vi "ROI Entry Screen.vi"() -> ()   [LabVIEW 2017]
uses:
  Typedefs/Line draw mode.ctl
  Typedefs/Top level VI states.ctl
  ROI Entry screen/Typedefs/ROI move buttons.ctl
  ROI Entry screen/Typedefs/ROI move mode.ctl
  Typedefs/Offsets cluster.ctl
  Typedefs/ROI management FG states.ctl
  ROI Entry screen/SubVIs/Automatic POI detection/Typedefs/Duplicate POI function enum.ctl
  Typedefs/Read Write Enum.ctl
  ROI Entry screen/Typedefs/ROI entry screen ctrl refs cluster.ctl
  Global Variables/General Globals.vi
  User profiles code/Globals/gl_UsrProfiles globals.vi
  ROI Entry screen/Globals/gl_ROI Entry UI globals.vi
  ROI Entry screen/Typedefs/ROI input mode.ctl
panel:
  out "Current ROI Type":string
  out "AOL Z ind. (um)":dbl caption="Motor Z" format="AOL Z   =  %#_g µm"
  in  "Load Reference Image":bool
  out "# POI":i32 format="%.0f ROI"
  in  "Max Z Proj":bool
  out "ROI":T1
  out "Number of lines left":i32 format="%.0f number of lines left"
  in  "Palette Type":T2(ring)
  out "Zplane ind":i32 caption="Z-Plane" format="Z-Plane %.0f"
  in  "Z-Plane Selector":i32(c297)=7
  out "Image Display":T3(plugin-control)
  out "Motor Z ind. (um)":dbl caption="Motor Z" format="Motor Z = %#_g µm"
  out "# of planes":i32 format="# of Planes = %.0f"
  in  "Intensity slider":cluster{i16, i16}(slide)={0, 4095} caption="Intensity" scale=0.0..4095.0
  in  "Z-stack folder path":path caption="Experiment folder path"
  in  "Channel":enum16{"Green", "Red"}(ring)
  in  "Enable cool-down time":bool caption="Enable stimulus"
  in  "Cool-down time (s)":dbl caption="Cool-down time" min=0.0 max=60.0 step=0.05 format="%#.2f s"
  in  "Enable funct. stimulus":bool caption="Enable stimulus"
  in  "Funct stim.trig.delay (sec)":dbl=0.5 caption="Stimulus trigger delay" min=0.0 max=60.0 step=0.001 format="%#.3fs"
  in  "ROI move mode":T4
  in  "ROI offset arrows":T5
  in  "Trial Length (sec)":dbl=1.0 caption="Trial Length" min=0.05 max=60.0 step=1.0 format="%#.3f s"
  in  "Arb Plane Entry":bool caption="Load\nolder\nPOI"
  in  "Load ROI File":bool caption="Load\nolder\nPOI"
  in  "POI Density":dbl(slide) scale=0.01..1.0
  in  "Auto Generate":bool
  in  "Equal size":bool=TRUE
  in  "Whole plane":bool
  in  "Zoom":dbl=1.0 min=0.001 max=10.0 step=0.1 format="%#.2f x"
  out "Next State":T6=enum."Live Imaging-START"
  in  "Scan dwell time per pixel (us)":dbl=0.1 caption="Scan dwell time\nper pixel (us)" min=0.05 max=20.0 step=0.01 format="%.2f"
  in  "POI dwell time (us)":dbl=4.0 caption="POI dwell time" min=0.05 max=20.0 format="%_3g µs"
  in  "Live Imaging":bool
  in  "Acquisition":bool
  in  "Line Mode":T7=enum."Orthogonal"
  in  "Number of Trials":u16=1 min=1 max=1000 format="%.0f trials"
  in  "Wavelength (nm)":dbl=920.0 caption="Wavelength" min=800.0 max=1080.0 step=1.0 format="%#_g nm"
  in  "Done/Close":bool
  in  "Clear Last":bool
  in  "Clear All":bool
  in  "POISelect Array":cluster{"System Array":dbl[], "Boolean":bool}[](array[cluster])
  in  "Step size (µm)":u8(slide)=1 min=1 max=100 step=1 scale=1.0..30.0
  # "ROI Removal"
  # "ROI Input"
  # "ROI AutoGen"
  # "Min"
  # "Max"
  # "Stimulus trigger delay"
  # "Cool-down time"
  # "ROI Offset"
  # "Settings"
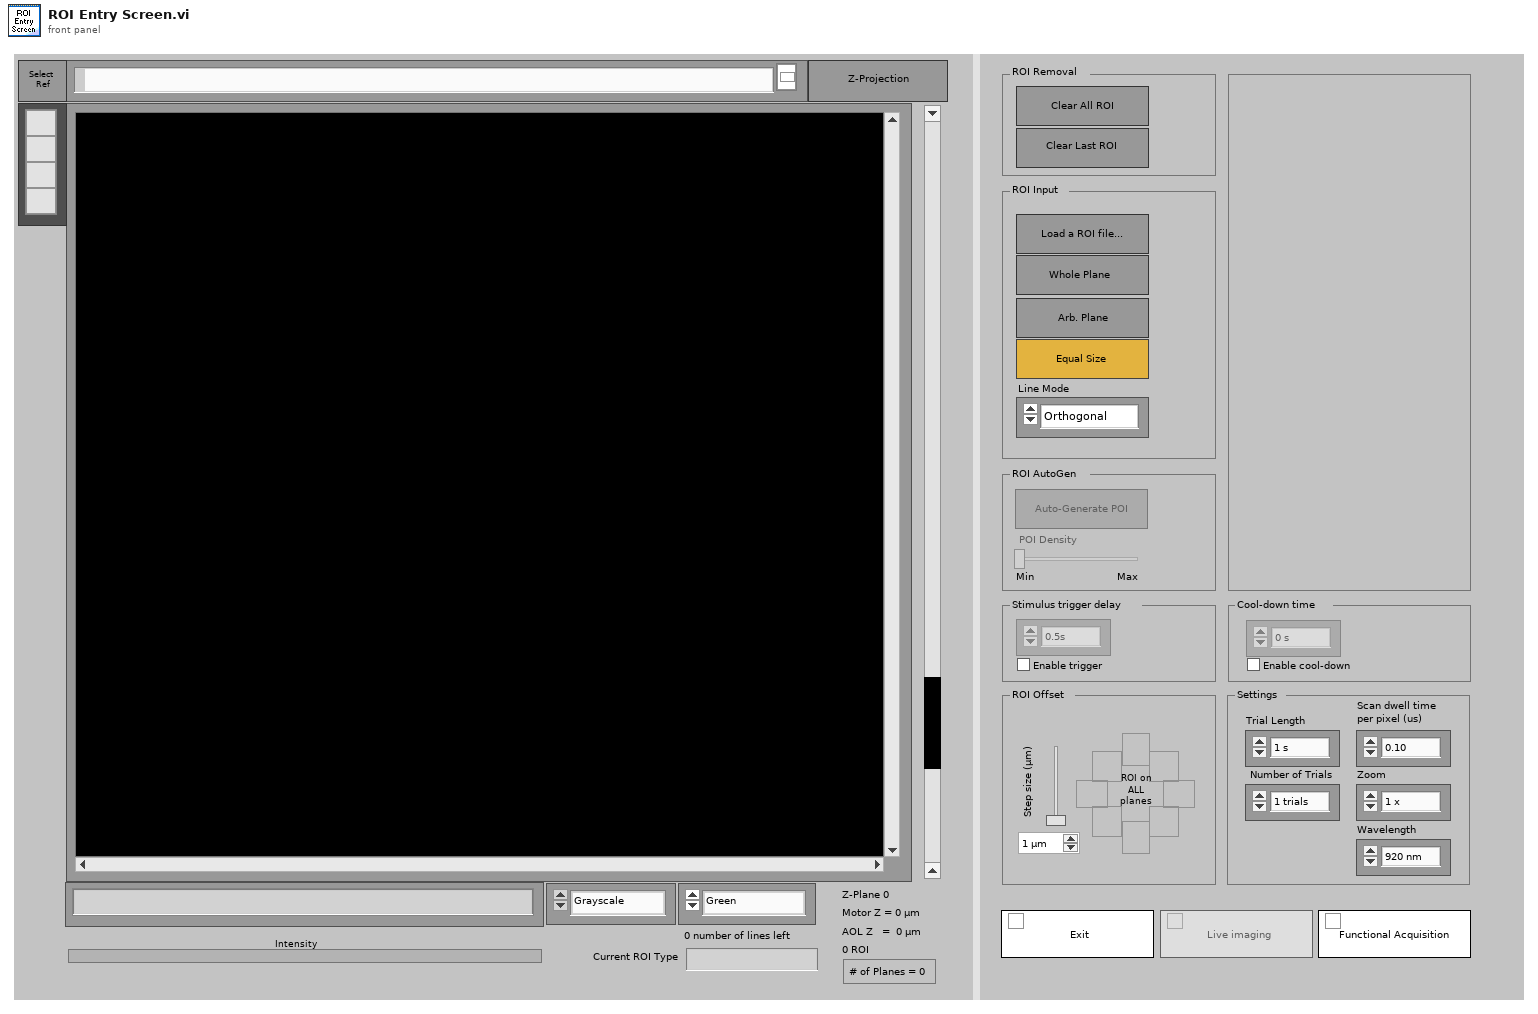
[diagram p1: front panel]
types:
  T1 = cluster{"Global Rectangle":i32[], "Contours":cluster{"Contour Type":u32, "ROI Type":u32, "Points":i32[]}[]}
  T2 = enum16{"Grayscale", "Binary", "Gradient", "Rainbow", "Temperature", "User Defined"}
  T3 = typedef "IMAQ Image.ctl" = refnum<image>
  T4 = typedef "ROI move mode.ctl" = enum16{"ROI on ALL planes", "ROI on current plane"}
  T5 = typedef "ROI move buttons.ctl" = cluster{"Right":bool, "Left":bool, "Up":bool, "Down":bool, "Up-left":bool, "Up-right":bool, "Down-left":bool, "Down-right":bool}
  T6 = typedef "Top level VI states.ctl" = enum16{"None", "Initialise UI", "<STACK PROTOCOL STATES>", "AOL Zstack-START", "AOL Zstack-STOP", "Motor Zstack-START", "Motor Zstack-STOP", "<ACQUISITION PROTOCOL STATES> ", "Functional Acquisition-START", "Functional Acquisition-STOP", "Single Plane Acquisition-START", "Single Plane Acquisition-STOP", "Volume Acquisition-START", "Volume Acquisition-STOP", "<LIVE IMAGING PROTOCOL STATES>", "Live Imaging-START", "Live Imaging-STOP", "Live Plane Imaging-START", "Live Plane Imaging-STOP", "Live Volume Imaging-START", "Live Volume Imaging-STOP", "<MOVEMENT CORRECTION PROTOCOL STATES>", "EXIT"}
  T7 = typedef "Line draw mode.ctl" = enum16{"Free draw", "Orthogonal"}
  T8 = typedef "Offsets cluster.ctl" = cluster{"X offset":i8, "Y offset":i8}
  T9 = cluster{"Load experiment data":refnum<user-event>, "Finish rectangle editing":refnum<user-event>, "Offset all ROI":refnum<user-event>}
  T10 = typedef "ROI info cluster.ctl" = cluster{"Global Rectangle":i32[], "Contours":cluster{"Contour Type":u32, "ROI Type":u32, "Points":i32[]}[]}
  T11 = typedef "ROI management FG states.ctl" = enum16{"Read", "Write", "Write-from dataset", "Clear Last", "Clear All", "Update ROIs time", "Reload last ROI set", "Offset all ROI", "Offset visible ROI"}
  T12 = typedef "ROI input mode.ctl" = enum16{"Unspecified", "Point-Line-Plane", "Volume"}
  T13 = enum8{"Enabled", "Disabled", "Disabled and Grayed Out"}
  T14 = typedef "Duplicate POI function enum.ctl" = enum16{"Generate", "Adjust number of POI", "Clear register"}
  T15 = typedef "Read Write Enum.ctl" = enum16{"Read", "Write"}
  T16 = typedef "ROI entry screen ctrl refs cluster.ctl" = cluster{"Done button":refnum<vi>, "Imaging button":refnum<vi>, "Acquisition button":refnum<vi>, "POI dwell time (us)":refnum<vi>, "Scan dwell time per pixel (us)":refnum<vi>, "# of planes":refnum<vi>, "Zoom Ctrl":refnum<vi>, "Equal size":refnum<vi>, "Channel":refnum<vi>, "Image Display":refnum<vi>, "Z-Plane Selector":refnum<vi>, "Number of lines left":refnum<vi>, "Z-stack folder path":refnum<vi>, "POI Density":refnum<vi>, "Arb Plane Entry":refnum<vi>, "Whole plane":refnum<vi>, "Clear Last":refnum<vi>, "Clear All":refnum<vi>, "Trial Length (sec)":refnum<vi>, "Palette Type":refnum<vi>, "Intensity slider":refnum<vi>, "# POI":refnum<vi>, "Max Z Proj":refnum<vi>, "Zplane ind":refnum<vi>, "Wavelength (nm)":refnum<vi>, "Number of Trials":refnum<vi>, "Funct stim.trig.enable":refnum<vi>, "Funct stim.trig.delay (s)":refnum<vi>, "Line Mode":refnum<vi>, "Step size (µm)":refnum<vi>, "ROI move mode":refnum<vi>, "Cool-down time (s)":refnum<vi>, "Enable cool-down time":refnum<vi>, "Motor Z ind. (um)":refnum<vi>, "AOL Z ind. (um)":refnum<vi>, "Load Reference Image":refnum<vi>, "SubPanel Call":refnum<vi>}
  T17 = typedef "ROI ID Enum.ctl" = enum16{"Point", "MiniScan", "Comp. MiniScan", "Rectangle", "Comp. volume", "Arb. plane point", "None"}
  T18 = typedef "lveventtype.ctl" = enum32{"Null", "Timeout", "Annotation Menu Selection", "Annotation Menu Selection?", "App Instance Close", "App Instance Close?", "Autoscale Range Change", "Bookmark Info Change", "Cell Edit", "Cell Edit?", "Cursor Grab", "Cursor Grab?", "Cursor Menu Selection", "Cursor Menu Selection?", "Cursor Move", "Cursor Release", "Data Change", "Direction Change", "Display State Change", "Drag Ended", "Drag Enter", "Drag Leave", "Drag Over", "Drag Source Update", "Drag Starting", "Drag Starting?", "Drop", "Exec State Change", "Key Down", "Key Down?", "Key Repeat", "Key Repeat?", "Key Up", "Listbox Double Click", "Menu Activation?", "Menu Selection (App)", "Menu Selection? (App)", "Menu Selection (User)", "Mouse Down", "Mouse Down?", "Mouse Enter", "Mouse Leave", "Mouse Move", "Mouse Up", "Mouse Wheel", "NI Security User Change (App)", "Pane Size", "Panel Close", "Panel Close?", "Panel Resize", "Plot Attribute Change", "Scale Range Change", "Shortcut Menu Activation?", "Shortcut Menu Selection (App)", "Shortcut Menu Selection? (App)", "Shortcut Menu Selection (User)", "Tree Double Click", "Tree Drag", "Tree Drag?", "Tree Drop", "Tree Drop?", "Tree Item Close", "Tree Item Close?", "Tree Item Open", "Tree Item Open?", "User Event", "Value Change"}
  T19 = typedef "ROI Entry screen VI interface 1.ctl" = cluster{"Last Image Display Event info":T20, "ROIs Info []":T21[], "Cancelled":bool, "Done button disabled?":enum8{"Enabled", "Disabled", "Disabled and Grayed Out"}, "Acquisition button disabled?":enum8{"Enabled", "Disabled", "Disabled and Grayed Out"}}
  T20 = typedef "Last Image Display Event info.ctl" = cluster{"Type":i32, "Tool":i32, "Coordinates":i32[], "Other Parameters":sgl[]}
  T21 = typedef "ROI spec.ctl" = cluster{"Coordinates":i32[], "Zoom":dbl, "ROI Enum":T17, "Z planeIdx(s)":i32[], "Z planecodes(s)":u8[], "Z start":dbl, "Z stop":dbl}
  T22 = typedef "ROI parameters data type.ctl" = cluster{"ROI index":dbl, "ROI ID":dbl, "ROI Time (ns)":dbl, "Pixels in ROI":dbl, "X start":dbl, "Y start":dbl, "Z start":dbl, "X stop":dbl, "Y stop":dbl, "Z stop":dbl, "Angle (deg)":dbl, "Composite ID":dbl, "Number of lines":dbl, "Frame Size":dbl, "Zoom":dbl, "Laser Power (%)":dbl, "ROI group ID":dbl, "Z Plane Idx":i32[], "Z Plane codes":i32[]}
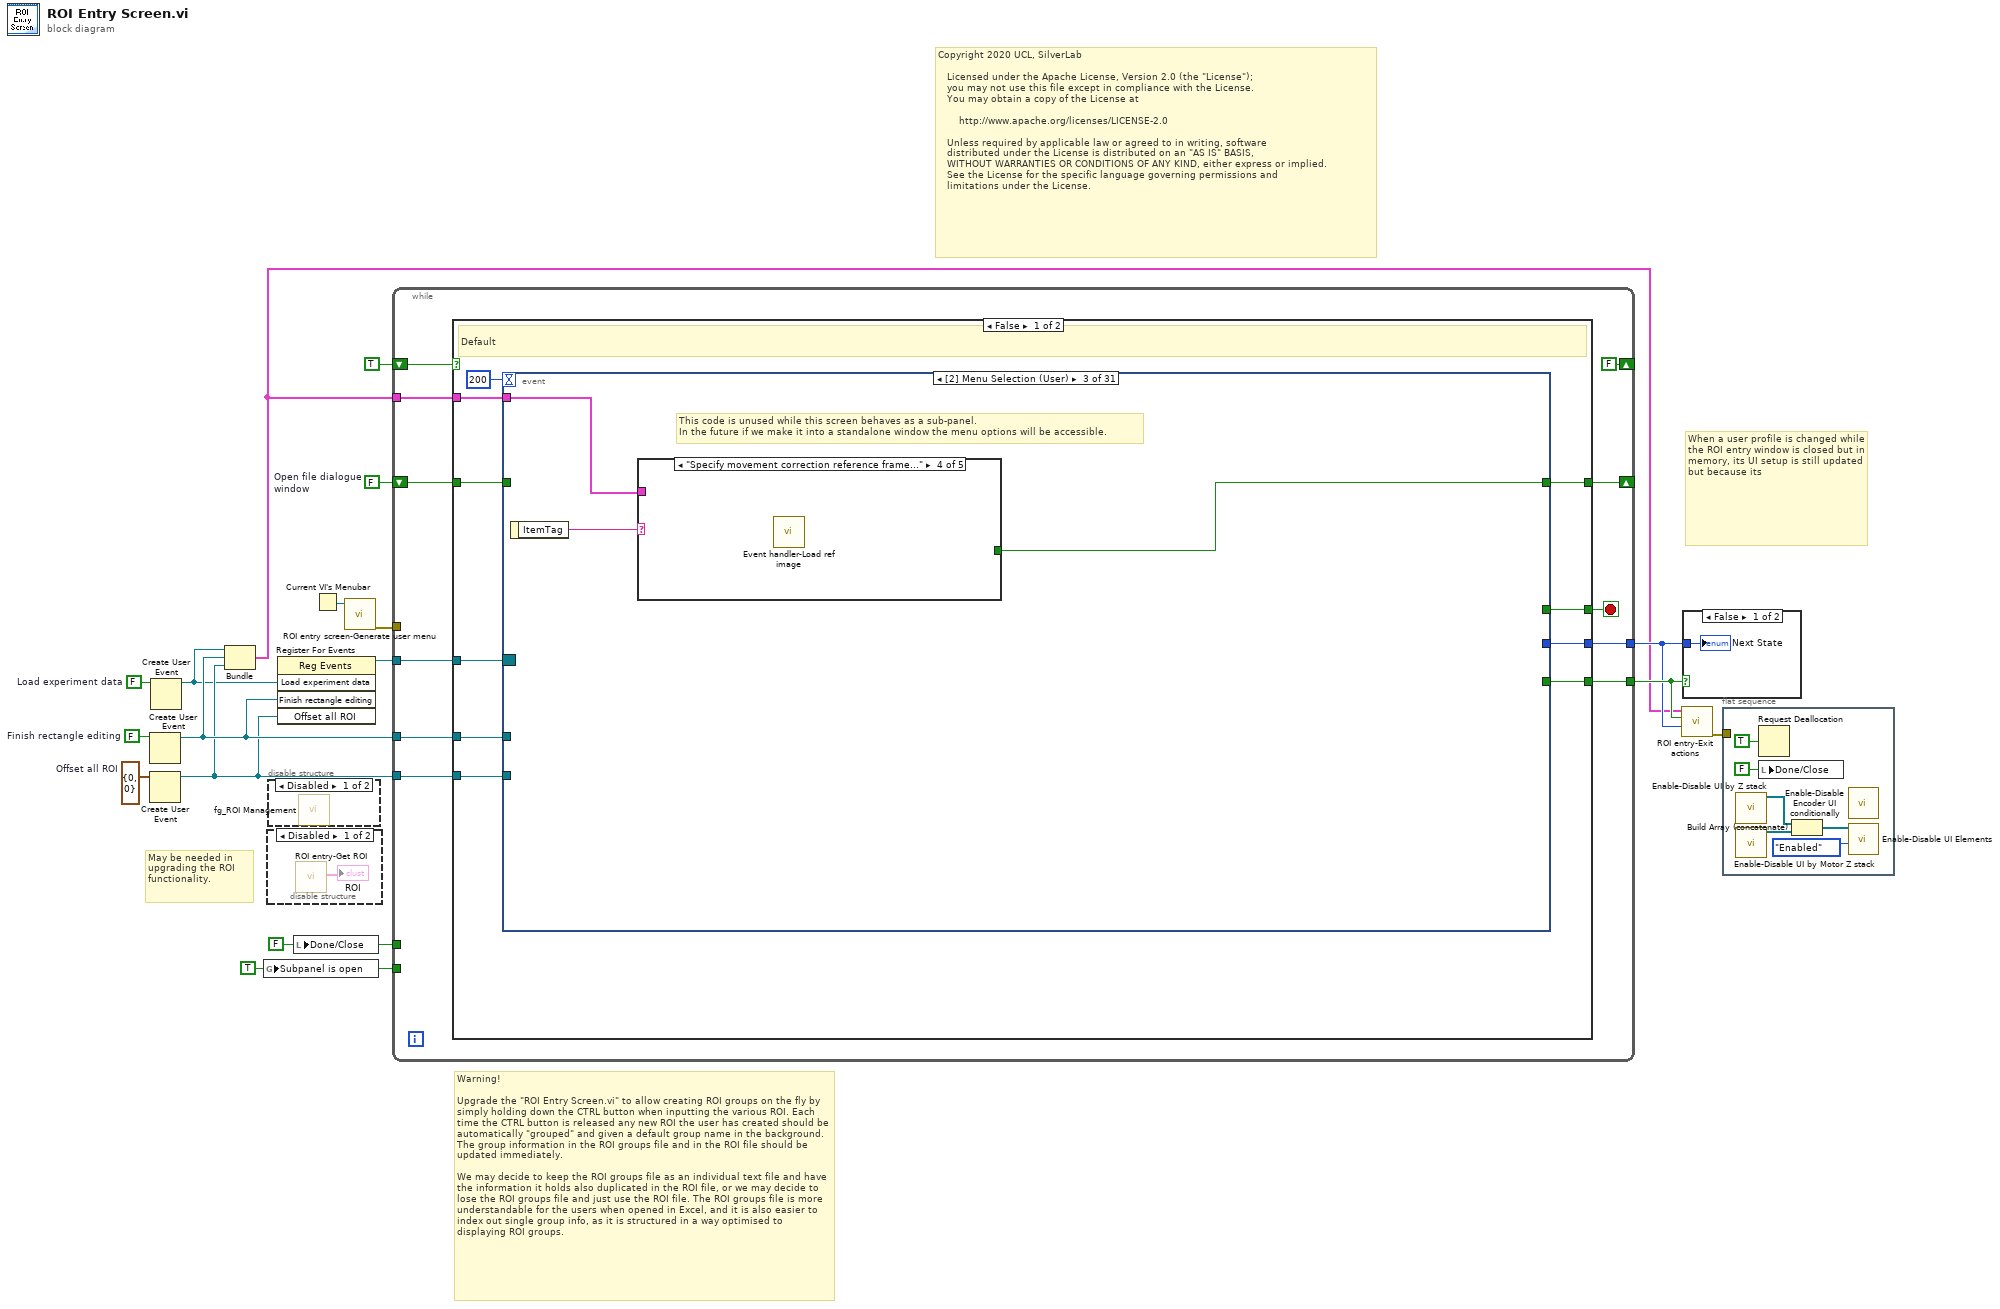
[diagram p0: block diagram]
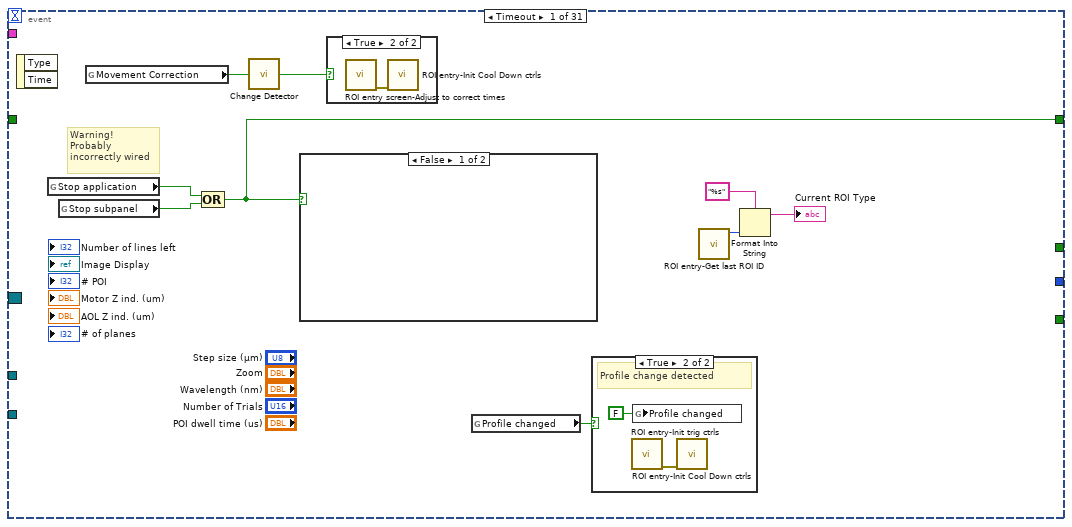
[diagram p5: hidden frame]
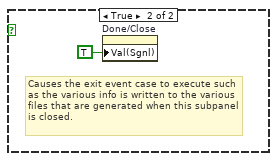
[diagram p8: hidden frame]
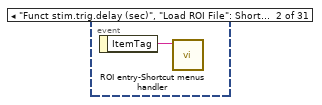
[diagram p9: hidden frame]
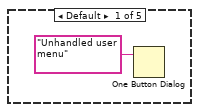
[diagram p10: hidden frame]
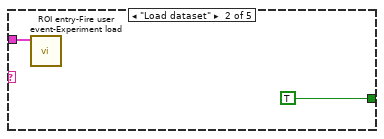
[diagram p11: hidden frame]
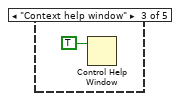
[diagram p12: hidden frame]
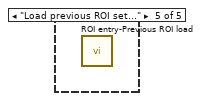
[diagram p13: hidden frame]
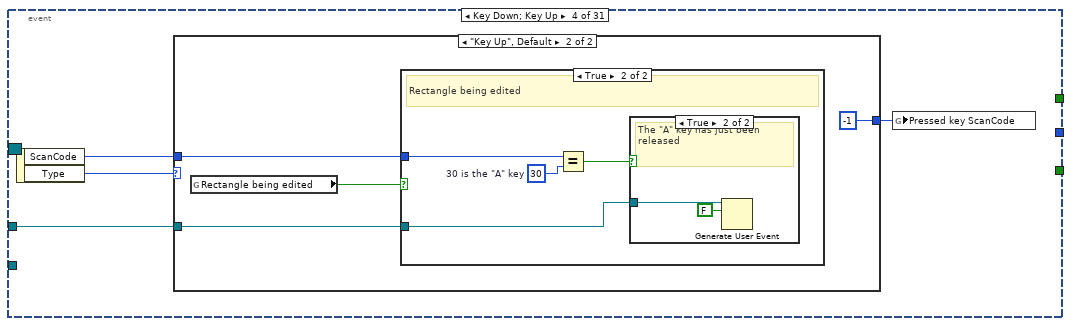
[diagram p14: hidden frame]
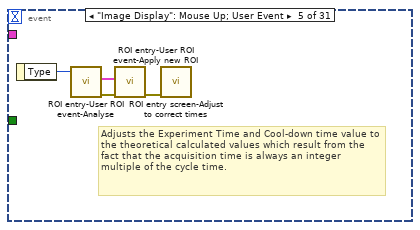
[diagram p18: hidden frame]
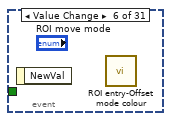
[diagram p19: hidden frame]
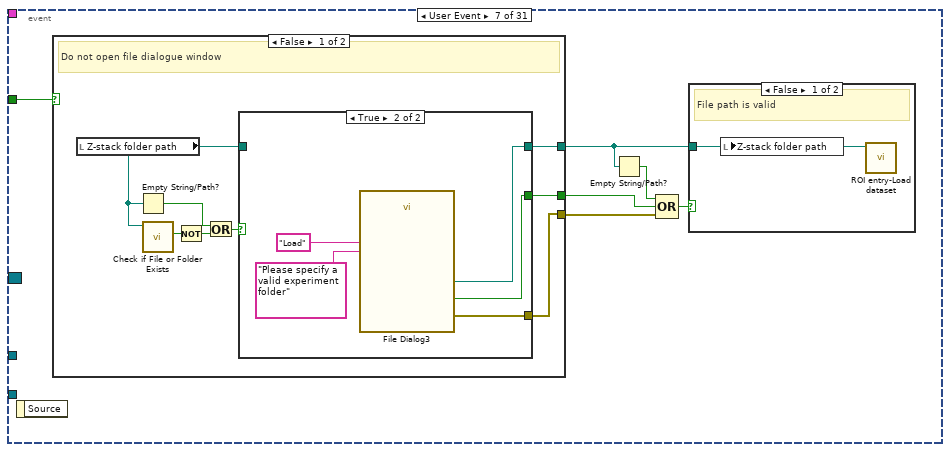
[diagram p20: hidden frame]
diagram:
  w5 = T8 {"X offset"=0, "Y offset"=0}  # Offset all ROI
  w6 = FALSE ("Done/Close")
  w12 = FALSE  # Finish rectangle editing
  w14 = TRUE ("Subpanel is open")
  w15 = FALSE  # Open file dialogue window
  w17 = FALSE  # Load experiment data
  # "Copyright 2020 UCL, SilverLab\n \n   Licensed under the Apache License, Version 2.0 (the \"License\");\n   you may not use this file except in compliance with the License.\n   You may obtain a copy of the License at\n \n       http://www.apache.org/licenses/LICENSE-2.0\n \n   Unless required by applicable law or agreed to in writing, software\n   distributed under the License is distributed on an \"AS IS\" BASIS,\n   WITHOUT WARRANTIES OR CONDITIONS OF ANY KIND, either express or implied.\n   See the License for the specific language governing permissions and\n   limitations under the License."
  # "When a user profile is changed while the ROI entry window is closed but in memory, its UI setup is still updated but because its"
  # "Warning!\n\nUpgrade the \"ROI Entry Screen.vi\" to allow creating ROI groups on the fly by simply holding down the CTRL button when inputting the various ROI. Each time the CTRL button is released any new ROI the user has created should be automatically \"grouped\" and given a default group name in the background. The group information in the ROI groups file and in the ROI file should be updated immediately.\n\nWe may decide to keep the ROI groups file as an individual text file and have the information it holds also duplicated in the ROI file, or we may decide to lose the ROI groups file and just use the ROI file. The ROI groups file is more understandable for the users when opened in Excel, and it is also easier to index out single group info, as it is structured in a way optimised to displaying ROI groups."
  # "May be needed in upgrading the ROI functionality."
  n1 = Create User Event(user event datatype=w12) -> (user event=w4:refnum<user-event>)  [unwired: 1 in, 1 out]
  n2 = Create User Event(user event datatype=w5) -> (user event=w3:refnum<user-event>)  [unwired: 1 in, 1 out]
  n3 = Create User Event(user event datatype=w17) -> (user event=w2:refnum<user-event>)  [unwired: 1 in, 1 out]
  n4 = Bundle("Load experiment data"=w2, "Finish rectangle editing"=w4, "Offset all ROI"=w3) -> (w1:T9)  [unwired: 1 in]
  n5 = global write "General Globals.vi" "Subpanel is open"(w14) -> ()
  n6 = disable-structure shown="Disabled" {
    frame Disabled {
      n7 = call "ROI entry-Get ROI.vi"() -> ("ROI info cluster (native format)"=→"ROI":T10)  [unwired: 10 in, 1 out]
    }
    frame Enabled {
    }
  }
  n8 = disable-structure shown="Disabled" {
    frame Disabled {
      n9 = call "fg_ROI Management.vi"() -> ()  [unwired: 6 in, 6 out]
    }
    frame Enabled {
    }
  }
  n10 = register-events(w2, w4, w3) -> (reference out=w16:refnum<event-registration>)  [unwired: 2 in, 1 out]
  n11 = local write "Done/Close"(w6) -> ()
  n12 = Current VI's Menubar() -> (w11:refnum<k9>)
  n13 = call "ROI entry screen-Generate user menu.vi"("Functional Viewer Menu in"=w11) -> ("error out"=w10:errorcluster)  [unwired: 9 in, 1 out]
  n14 = while {
    shift-right: [FALSE] -> _
    shift-left: TRUE -> [w28]
    tunnel: [w26] -> w8
    tunnel: w16 -> [w25]
    tunnel: w1 -> [w24]
    shift-right: [w23] -> _
    shift-left: w15 -> [w22]
    tunnel: w14 -> [_]
    tunnel: w4 -> [w21]
    tunnel: w10 -> [_]
    tunnel: [w20] -> w9
    tunnel: w6 -> [_]
    tunnel: w3 -> [w19]
    stop <- w29 stop-if-true
    n15 = case shown="False" w28 {
      tunnel: [w38 _] -> w29
      tunnel: [w37 _] -> w26
      tunnel: w25 -> [w36 _]
      tunnel: w24 -> [w35 w282]
      tunnel: [w33 w283] -> w23
      tunnel: w22 -> [w34 _]
      tunnel: w21 -> [w32 _]
      tunnel: [w31 _] -> w20
      tunnel: w19 -> [w30 _]
      frame False {
        # "Default"
        n16 = event shown="[2] Menu Selection (User)" {
          selector: w36 -> [_ _ _ _ _ _ _ _ _ _ _ _ _ _ _ _ _ _ _ _ _ _ _ _ _ _ _ _ _ _ _]
          dyn-events: _ -> [_ _ _ _ _ _ _ _ _ _ _ _ _ _ _ _ _ _ _ _ _ _ _ _ _ _ _ _ _ _ _]
          timeout: 200 -> [_ _ _ _ _ _ _ _ _ _ _ _ _ _ _ _ _ _ _ _ _ _ _ _ _ _ _ _ _ _ _]
          tunnel: [_ _ _ _ _ _ _ _ _ _ _ _ _ _ _ _ _ _ _ _ _ _ _ _ w257 _ _ _ _ _ w280] -> w38
          tunnel: [_ _ _ _ _ _ _ _ _ _ _ _ _ _ _ _ _ _ _ _ _ _ _ _ w258 _ _ _ _ _ _] -> w37
          tunnel: w35 -> [_ _ w55 _ _ _ _ _ _ _ _ w162 _ _ _ _ _ _ _ _ _ _ _ _ _ _ _ _ _ _ _]
          tunnel: w34 -> [_ _ _ _ _ _ w84 _ _ w158 _ _ _ _ _ _ _ _ _ _ _ _ _ _ _ _ _ _ _ _ _]
          tunnel: [w47 _ w54 _ _ _ _ _ _ _ _ _ _ _ _ _ _ _ _ _ _ _ _ _ _ _ _ _ _ _ _] -> w33
          tunnel: w32 -> [_ _ _ w64 _ _ _ _ _ _ _ _ _ _ _ _ _ _ _ _ _ _ _ _ _ _ _ _ _ _ _]
          tunnel: [_ _ _ _ _ _ _ _ _ _ _ _ _ _ _ _ _ _ _ _ _ _ _ _ _ _ _ _ _ _ w280] -> w31
          tunnel: w30 -> [_ _ _ _ _ _ _ _ w157 _ _ _ _ _ _ _ _ _ _ _ _ _ _ _ _ _ _ _ _ _ _]
          event Timeout {
            # "Warning!\nProbably\nincorrectly wired"
            n17 = event-data() -> ()  [unwired: 1 in, 2 out]
            n18 = global read "General Globals.vi" "Stop application"() -> (w48:bool)
            n19 = global read "General Globals.vi" "Stop subpanel"() -> (w46:bool)
            n20 = global read "General Globals.vi" "Movement Correction"() -> (w45:bool)
            n21 = Compound Arithmetic op=OR(w48, w46) -> (w47:bool)
            n22 = call <userlib>:"Change Detector.vi"("Value"=w45) -> ("Changed?"=w44:bool)
            n23 = case shown="False" w47 {
              frame False {
              }
              frame True {
                # "Causes the exit event case to execute such as the various info is written to the various files that are generated when this subpanel is closed."
                n24 = property on="Done/Close" class="Bool (strict)"("Val(Sgnl)"=TRUE) -> ()  [unwired: 2 in, 2 out]
              }
            }
            n25 = case shown="True" w44 {
              frame False {
              }
              frame True {
                n26 = call "ROI entry screen-Adjust to correct times.vi"() -> ("error out"=w51:errorcluster)  [unwired: 10 in, 1 out]
                n27 = call "ROI entry-Init Cool Down ctrls.vi"("error in (no error)"=w51) -> ()  [unwired: 10 in, 1 out]
              }
            }
            n28 = global read "gl_UsrProfiles globals.vi" "Profile changed"() -> (w43:bool)
            n29 = case shown="True" w43 {
              frame False {
                # "Idle"
              }
              frame True {
                # "Profile change detected"
                n30 = call "ROI entry-Init trig ctrls.vi"() -> ("error out"=w50:errorcluster)  [unwired: 11 in]
                n31 = global write "gl_UsrProfiles globals.vi" "Profile changed"(FALSE ("Profile changed")) -> ()
                n32 = call "ROI entry-Init Cool Down ctrls.vi"("error in (no error)"=w50) -> ()  [unwired: 10 in, 1 out]
              }
            }
            n33 = call "ROI entry-Get last ROI ID.vi"() -> ("ROI ID Enum"=w42:T17)  [unwired: 8 in, 3 out]
            n34 = Format Into String(format string="%s", w42) -> (resulting string=→"Current ROI Type":string)  [unwired: 2 in, 1 out]
          }
          event "Funct stim.trig.delay (sec)", "Load ROI File": Shortcut Menu Selection (User) {
            n35 = event-data() -> ("ItemTag"=w53:string)  [unwired: 1 in]
            n36 = call "ROI entry-Shortcut menus handler.vi"("ItemTag"=w53) -> ()  [unwired: 11 in]
          }
          event Menu Selection (User) {
            # "This code is unused while this screen behaves as a sub-panel.\nIn the future if we make it into a standalone window the menu options will be accessible."
            n37 = event-data() -> ("ItemTag"=w56:string)  [unwired: 1 in]
            n38 = case shown="\"Specify movement correction reference frame...\"" w56 {
              tunnel: w55 -> [_ w58 _ _ _]
              tunnel: [_ TRUE _ _ _] -> w54
              frame Default {
                n39 = One Button Dialog(message="Unhandled user menu") -> ()  [unwired: 1 in, 1 out]
              }
              frame "Load dataset" {
                n40 = call "ROI entry-Fire user event-Experiment load.vi"("User Events Cluster"=w58) -> ()  [unwired: 10 in, 1 out]
              }
              frame "Context help window" {
                n41 = Control Help Window(1:TRUE ("Show")) -> ()  [unwired: 1 in]
              }
              frame "Specify movement correction reference frame..." {
                n42 = call "Event handler-Load ref image.vi"() -> ()  [unwired: 10 in, 2 out]
              }
              frame "Load previous ROI set..." {
                n43 = call "ROI entry-Previous ROI load.vi"() -> ()  [unwired: 11 in, 1 out]
              }
            }
          }
          event Key Down; Key Up {
            n44 = event-data() -> ("ScanCode"=w63:i16, "Type"=w62:T18)  [unwired: 1 in]
            n45 = case shown="\"Key Up\", Default" w62 {
              tunnel: w64 -> [_ w69]
              tunnel: w63 -> [w65 w68]
              tunnel: [w65 i16 -1 ("ScanCode")] -> w61
              frame "Key Down" {
              }
              frame "Key Up", Default {
                n46 = global read "gl_ROI Entry UI globals.vi" "Rectangle being edited"() -> (w67:bool)
                n47 = case shown="True" w67 {
                  tunnel: w68 -> [_ w72]
                  tunnel: w69 -> [_ w71]
                  frame False {
                  }
                  frame True {
                    w73 = i16 30  # 30 is the "A" key
                    # "Rectangle being edited"
                    n48 = Equal?(x=w72, y=w73) -> (x = y?=w70:bool)
                    n49 = case shown="True" w70 {
                      tunnel: w71 -> [_ w75]
                      frame False {
                      }
                      frame True {
                        # "The \"A\" key has just been released"
                        n50 = Generate User Event(user event=w75, event data cluster=FALSE ("event data")) -> ()  [unwired: 2 in, 2 out]
                      }
                    }
                  }
                }
              }
            }
            n51 = global write "gl_ROI Entry UI globals.vi" "Pressed key ScanCode"(w61) -> ()
          }
          event "Image Display": Mouse Up; User Event {
            # "Adjusts the Experiment Time and Cool-down time value to the theoretical calculated values which result from the fact that the acquisition time is always an integer multiple of the cycle time."
            n52 = event-data() -> ("Type"=w79:u32)  [unwired: 1 in]
            n53 = call "ROI entry-User ROI event-Analyse.vi"("Event Type"=w79) -> ("error out"=w77:errorcluster, "output cluster"=w78:T19)  [unwired: 9 in]
            n54 = call "ROI entry-User ROI event-Apply new ROI.vi"("error in (no error)"=w77, "Input cluster"=w78) -> ("error IO"=w76:errorcluster)  [unwired: 9 in]
            n55 = call "ROI entry screen-Adjust to correct times.vi"("error in (no error)"=w76) -> ()  [unwired: 9 in, 2 out]
          }
          event Value Change {
            n56 = event-data() -> ()  [unwired: 1 in, 1 out]
            n57 = call "ROI entry-Offset mode colour.vi"() -> ()  [unwired: 11 in, 1 out]
          }
          event User Event {
            n58 = event-data() -> ()  [unwired: 1 in, 1 out]
            n59 = case shown="False" w84 {
              tunnel: [w88 w103] -> w85
              tunnel: [w86 w102] -> w83
              tunnel: [w87 w101] -> w82
              frame False {
                # "Do not open file dialogue window"
                n60 = local read "Z-stack folder path"() -> (w89:path)
                n61 = Empty String/Path?(string/path=w89) -> (empty?=w93:bool)
                n62 = call <vilib>:"Check if File or Folder Exists.vi"("path"=w89) -> ("file or folder exists?"=w91:bool)  [unwired: 8 in, 2 out]
                n63 = Not(x=w91) -> (.not. x?=w92:bool)
                n64 = Or(x=w93, y=w92) -> (x .or. y?=w90:bool)
                n65 = case shown="True" w90 {
                  tunnel: w89 -> [w94 _]
                  tunnel: [w94 w98] -> w88
                  tunnel: [_ w97] -> w87
                  tunnel: [_ w96] -> w86
                  frame False {
                  }
                  frame True {
                    n66 = call "File Dialog3"("prompt"="Please specify a valid experiment folder", "button label"="Load") -> ("selected path"=w98:path, "cancelled"=w96:bool, "error out"=w97:errorcluster)  [unwired: 10 in, 1 out]
                  }
                }
              }
              frame True {
                # "Open file dialogue window"
                n67 = call "File Dialog2"("prompt"="Please specify a valid experiment folder", "button label"="Load") -> ("selected path"=w103:path, "cancelled"=w102:bool, "error out"=w101:errorcluster)  [unwired: 10 in, 1 out]
              }
            }
            n68 = Empty String/Path?(string/path=w85) -> (empty?=w81:bool)
            n69 = Compound Arithmetic op=OR(w81, w83, w82) -> (w80:bool)
            n70 = case shown="False" w80 {
              tunnel: w85 -> [w105 _]
              frame False {
                # "File path is valid"
                n71 = local write "Z-stack folder path"(w105) -> ()
                n72 = call "ROI entry-Load dataset.vi"("Experiment folder path OR Z-stack folder path"=w105) -> ()  [unwired: 10 in, 1 out]
              }
              frame True {
                # "Empty file path / Not a path / User cancelled / Error"
              }
            }
          }
          event User Event {
            n73 = event-data() -> ("X offset"=w107:i8, "Y offset"=w106:i8)  [unwired: 1 in]
            n74 = disable-structure shown="Disabled" {
              disable-tunnel: w107 -> [_ w155]
              disable-tunnel: w106 -> [_ w154]
              frame Disabled {
                w108 = 0.0  # Y Offset
                w109 = 0.0  # X Offset
                # "WARNING!\nOld functionality.\nMust be upgraded for rig 3."
                n75 = call "POISelection.vi"("POISelectArrayIn"="POISelect Array") -> ("POI array"=w125:dbl[][])  [unwired: 9 in, 1 out]
                n76 = Index Array(array=w125, index (col) #1=1 ("index (row)"), index (col) #2=2 ("index (col)")) -> (element #1=w126:dbl[], element #2=w118:dbl[])  [unwired: 2 in]
                n77 = Add(x=w126, y=w109) -> (x+y=w124:dbl[])
                n78 = Add(x=w118, y=w108) -> (x+y=w117:dbl[])
                n79 = Replace Array Subset(array=w125, new element #1=w124, index (col) #1=1 ("disabled index (col)"), new element #2=w117, index (col) #2=2 ("index (col)")) -> (w120:dbl[][])  [unwired: 2 in]
                n80 = call "ROI entry-Get selected Z-plane index.vi"() -> ("Z-plane selector (index)"=w110:i32)  [unwired: 10 in, 1 out]
                n81 = call "ROI entry-Get Max Proj setting.vi"() -> ("Max Z-projection setting's value"=w111:bool)  [unwired: 10 in, 1 out]
                n82 = call "ROI entry-Clear ROI overlay.vi"() -> ("error out"=w113:errorcluster, "Image Out"=w114:T3)  [unwired: 10 in]
                n83 = for {
                  tunnel: w120 -> [w133] mode=indexing
                  shift-right: [w136] -> w112
                  shift-left: w114 -> [w135]
                  tunnel: w110 -> [w129]
                  tunnel: w113 -> [_]
                  tunnel: w111 -> [w127]
                  n84 = Index Array(array=w133, index=3) -> (element=w131:dbl)
                  n85 = Delete From Array(array=w133, index=0) -> (deleted portion=w128:dbl, array with subset deleted=w134:dbl[])  [unwired: 1 in]
                  n86 = Equal?(x=w131, y=w129) -> (x = y?=w130:bool)
                  n87 = case shown="True" w127 {
                    tunnel: [w142 w153] -> w136
                    tunnel: w135 -> [w141 w152]
                    tunnel: w134 -> [w140 w151]
                    tunnel: w130 -> [w139 _]
                    tunnel: w128 -> [w138 w150]
                    frame False {
                      n88 = case shown="True" w139 {
                        tunnel: [w143 w148] -> w142
                        tunnel: w141 -> [w143 w147]
                        tunnel: w138 -> [_ w146]
                        tunnel: w140 -> [_ w144]
                        frame False {
                        }
                        frame True {
                          n89 = Increment(x=w146) -> (x+1=w145:dbl)
                          n90 = call "PointOverlayV1.vi"("Point"=w144, "Count"=w145, "Image1"=w147) -> ("Image1 Out"=w148:T3)  [unwired: 8 in]
                        }
                      }
                    }
                    frame True {
                      n91 = Increment(x=w150) -> (x+1=w149:dbl)
                      n92 = call "PointOverlayV1.vi"("Point"=w151, "Count"=w149, "Image1"=w152) -> ("Image1 Out"=w153:T3)  [unwired: 8 in]
                    }
                  }
                }
                n93 = call "POIConvert.vi"("POI array"=w120) -> ("POISelectArrayOut"=w123:cluster{"System Array":dbl[], "Boolean":bool}[])  [unwired: 10 in]
                n94 = local write "POISelect Array"(w123) -> ()
                n95 = call "ROI entry-Image display write.vi"("Value"=w112) -> ()  [unwired: 4 in, 1 out]
              }
              frame Enabled {
                n96 = call "ROI entry-Offset all ROI.vi"("Y offset"=w154, "X offset"=w155) -> ()  [unwired: 9 in, 1 out]
              }
            }
          }
          event Value Change {
            n97 = event-data() -> ("NewVal"=w156:T5)  [unwired: 1 in]
            n98 = call "ROI entry-Event handler-ROI offset.vi"("Offset all ROI-User Event in"=w157, "ROI offset arrows: NewVal"=w156) -> ()  [unwired: 9 in, 1 out]
          }
          event "Load ROI File": Value Change {
            # "Adjusts the Experiment Time and Cool-down time value to the theoretical calculated values which result from the fact that the acquisition time is always an integer multiple of the cycle time."
            n99 = event-data() -> ()  [unwired: 1 in, 1 out]
            n100 = flat-sequence {
              tunnel: [w160] -> w159
              tunnel: w158 -> [_]
              tunnel: w159 -> [_]
              frame #0 {
                n101 = call "ROI entry-Previous ROI load.vi"() -> ("Proceed"=w160:bool)  [unwired: 11 in]
              }
              frame #1 {
                n102 = call "ROI entry screen-Adjust to correct times.vi"() -> ()  [unwired: 10 in, 2 out]
              }
            }
          }
          event Value Change {
            n103 = event-data() -> ()  [unwired: 1 in, 1 out]
            n104 = call "fgv_ROI equal size line coords.vi"("Function"=enum16{"Intialize", "Write", "Read", "Clear"}."Clear") -> ()  [unwired: 9 in, 2 out]
          }
          event "Z-stack folder path": Value Change {
            n105 = event-data() -> ()  [unwired: 1 in, 1 out]
            n106 = call "ROI entry-Fire user event-Experiment load.vi"("User Events Cluster"=w162) -> ()  [unwired: 10 in, 1 out]
          }
          event "Z-Plane Selector": Value Change {
            w165 = FALSE ("Max Z Proj")
            # "Max Z-projection button automatically released when the scrollbar is moved."
            # "Compensates for Labview bug."
            n107 = event-data() -> ()  [unwired: 1 in, 1 out]
            n108 = property on="Z-Plane Selector" class="Scroll (strict)"() -> ("DocMax"=w171:dbl, "DocMin"=w170:dbl)  [unwired: 2 in, 2 out]
            n109 = feedback-in #1("Z-Plane Selector") -> ()
            n110 = feedback #1() -> (w172:i32)  [unwired: 1 in]
            n111 = Decrement(x=w171) -> (x-1=w166:dbl)
            n112 = property on="Z-Plane Selector" class="Scroll (strict)"() -> ("PageSize"=w164:dbl)  [unwired: 2 in, 2 out]
            n113 = local write "Max Z Proj"(w165) -> ()
            n114 = Less?(x="Z-Plane Selector", y=w170) -> (x < y?=w169:bool)
            n115 = Greater?(x="Z-Plane Selector", y=w166) -> (0:w168:bool)
            n116 = feedback #2() -> (w163:dbl)  [unwired: 1 in]
            n117 = feedback-in #2(w164) -> ()
            n118 = Or(x=w168, y=w169) -> (x .or. y?=w167:bool)
            n119 = case shown="False" w167 {
              tunnel: w172 -> [_ w178]
              tunnel: "Z-Plane Selector" -> [w174 _]
              tunnel: w165 -> [_ _]
              tunnel: w163 -> [_ w179]
              frame False {
                # "Input value is in range"
                n120 = flat-sequence {
                  tunnel: w174 -> [w175]
                  frame #0 {
                    "Zplane ind" <- w175
                  }
                  frame #1 {
                    n121 = call "ROI entry-Handle ROI change.vi"("ROI management"=ROI_management_FG_states."Read") -> ("error out"=w176:errorcluster)  [unwired: 8 in, 2 out]
                    n122 = call "ROI entry-Index Zplane position.vi"("error in (no error)"=w176) -> ()  [unwired: 9 in, 2 out]
                  }
                }
              }
              frame True {
                # "Prevents out of range inputs"
                n123 = property on="Z-Plane Selector" class="Scroll (strict)"("PageSize"=w179) -> ()  [unwired: 2 in, 2 out]
                n124 = call "ROI entry-Set Z-plane selector.vi"("Z-plane selector value"=w178) -> ()  [unwired: 10 in, 1 out]
              }
            }
          }
          event "Channel", "Max Z Proj": Value Change {
            n125 = event-data() -> ()  [unwired: 1 in, 1 out]
            n126 = call "ROI entry-Event handler-Max projection.vi"() -> ()  [unwired: 11 in, 1 out]
          }
          event "Intensity slider": Value Change {
            n127 = event-data() -> ()  [unwired: 1 in, 1 out]
            n128 = call "ROI entry-Set display mapping.vi"() -> ()  [unwired: 11 in, 1 out]
          }
          event "Palette Type": Value Change {
            n129 = event-data() -> ("NewVal"=w180:T2)  [unwired: 1 in]
            n130 = call "ROI entry-Set palette type.vi"("Palette:Palette Type"=w180) -> ()  [unwired: 10 in, 1 out]
          }
          event "Arb Plane Entry": Value Change {
            n131 = event-data() -> ()  [unwired: 1 in, 1 out]
            n132 = call "ROI entry-Event handler-Arb entry.vi"() -> ()  [unwired: 11 in, 1 out]
          }
          event "Whole plane": Value Change {
            n133 = event-data() -> ()  [unwired: 1 in, 1 out]
            n134 = call "ROI entry-Event handler-Whole plane.vi"() -> ()  [unwired: 12 in]
          }
          event "Equal size": Value Change {
            n135 = event-data() -> ()  [unwired: 1 in, 1 out]
            n136 = call "ROI entry-Event handler-Equal Size.vi"() -> ()  [unwired: 12 in]
          }
          event "Auto Generate": Value Change {
            n137 = event-data() -> ()  [unwired: 1 in, 1 out]
            n138 = disable-structure shown="Disabled" {
              frame Disabled {
                n139 = call "fg_ROI Management.vi"("Function"=ROI_management_FG_states."Read") -> ("ROI Setup"=w184:T22[])  [unwired: 5 in, 5 out]
                n140 = Empty Array?(array=w184) -> (empty?=w183:bool)
                n141 = case shown="False" w183 {
                  tunnel: [w203 w206] -> w182
                  frame False {
                    # "User-specified ROIs exist"
                    n142 = Two Button Dialog(message="WARNING\n\nThe Auto-generate function will overwrite existing ROIs.\n", 2:"Proceed..." ("T button name (\"OK\")")) -> (T button?=w203:bool)  [unwired: 1 in]
                  }
                  frame True {
                    w206 = TRUE  # Proceed
                    # "No user-specified ROIs"
                  }
                }
                n143 = case shown="True" w182 {
                  frame False {
                  }
                  frame True {
                    n144 = call "POI Autogen number entry window.vi"() -> ("Cancelled"=w185:bool, "Number of POI"=w186:i32)  [unwired: 10 in]
                    n145 = case shown="False" w185 {
                      tunnel: w186 -> [w198 _]
                      frame False {
                        w196 = TRUE
                        w201 = T13."Enabled" ("Disabled")
                        # "Not cancelled. Auto-generate POIs."
                        n146 = global read "gl_ROI Entry UI globals.vi" "ROI entry ctrl refs"() -> (w192:T16)
                        n147 = call "fg_ROI Management.vi"("Function"=ROI_management_FG_states."Clear All") -> ("error out"=w191:errorcluster)  [unwired: 5 in, 5 out]
                        n148 = call "ROI entry-Clear ROI overlay.vi"("error in (no error)"=w191) -> ("Image Out"=w190:T3)  [unwired: 9 in, 1 out]
                        n149 = Unbundle By Name(w192) -> ("Image Display"=w193:refnum<vi>)
                        n150 = call "Auto generate POIs.vi"("Number of POI to generate"=w198, "Image refnum in"=w190) -> ("POI Array"=w199:T21[], "Number of POI generated"=w200:i32)  [unwired: 8 in]
                        n151 = call "ROI entry-Get selected Z-plane index.vi"() -> ("Z-plane selector (index)"=w189:i32)  [unwired: 10 in, 1 out]
                        n152 = global write "gl_ROI Entry UI globals.vi" "Input Mode"(ROI_input_mode."Point-Line-Plane" ("t")) -> ()
                        n153 = Initialize Array(w189, w200) -> (w188:i32[])
                        n154 = property class="ImageControl"(reference=w193, "Line Tool Button Visible"=w196, "Point Tool Button Visible"=w196) -> ()  [unwired: 1 in, 2 out]
                        n155 = call "ROI entry screen-main buttons management.vi"("Acquisition button boolean text"="Functional Acquisition" ("Boolean Text.Text"), "Imaging button disabled?"=T13."Disabled and Grayed Out" ("Disabled"), "Acquisition button disabled?"=w201, "Done button disabled?"=w201) -> ()  [unwired: 8 in]
                        n156 = call "Apply ROIs.vi"("Mode (Redraw All)"=enum16{"Redraw All", "Draw Last"}."Redraw All", "ROIs Info []"=w199, 11:w188) -> ()  [unwired: 5 in, 4 out]
                      }
                      frame True {
                        # "Cancelled"
                      }
                    }
                  }
                }
              }
              frame Enabled {
                n157 = call "POI Gen Engine.vi"("Function"=Duplicate_POI_function_enum."Generate") -> ()  [unwired: 10 in, 1 out]
              }
            }
          }
          event "POI Density": Value Change {
            n158 = event-data() -> ()  [unwired: 1 in, 1 out]
            n159 = global read "General Globals.vi" "First autogen"() -> (w208:bool)
            n160 = case shown="False" w208 {
              frame False {
                n161 = call "POI Gen Engine.vi"("Function"=Duplicate_POI_function_enum."Adjust number of POI") -> ()  [unwired: 10 in, 1 out]
              }
              frame True {
              }
            }
          }
          event "Clear All": Value Change {
            n162 = event-data() -> ()  [unwired: 1 in, 1 out]
            n163 = call "ROI entry-Event handler-Clear All ROI.vi"() -> ()  [unwired: 12 in]
          }
          event "Clear Last": Value Change {
            # "WARNING!\nMore work may be needed"
            n164 = event-data() -> ()  [unwired: 1 in, 1 out]
            n165 = call "ROI entry-Get last ROI ID.vi"() -> ("error out"=w212:errorcluster, "NO ROI"=w211:bool, "ROI ID Enum"=w210:T17)  [unwired: 8 in, 1 out]
            n166 = call "ROI entry-Handle ROI change.vi"("error in (no error)"=w212, "ROI management"=ROI_management_FG_states."Clear Last" ("Function")) -> ("No ROI"=w214:bool, "Number of ROI"=w213:i32)  [unwired: 7 in, 1 out]
            n167 = case shown="False" w214 {
              tunnel: w213 -> [w216 _]
              tunnel: w211 -> [_ w220]
              tunnel: w210 -> [_ w219]
              frame False {
                # "Some ROI exist"
                n168 = local read "Arb Plane Entry"() -> (w217:bool)
                n169 = case shown="True" w217 {
                  tunnel: w216 -> [w218 _]
                  frame True {
                    # "Arb. Plane Entry mode is active"
                    n170 = call "ROI entry screen-Arb plane UI setup.vi"("Number of ROI"=w218) -> ()  [unwired: 11 in]
                  }
                  frame False {
                    # "Arb. Plane Entry mode is not active"
                  }
                }
              }
              frame True {
                # "No ROIs specified"
                n171 = case shown="False" w220 {
                  tunnel: w219 -> [w222 _]
                  frame False {
                    n172 = call "ROI entry-Set ROI tool on Clear All.vi"("Last ROI ID Enum"=w222) -> ()  [unwired: 10 in, 1 out]
                  }
                  frame True {
                  }
                }
                n173 = call "ROI entry-Actions on all ROI cleared.vi"("No ROIs (T)"=TRUE ("empty?")) -> ()  [unwired: 11 in]
              }
            }
          }
          event "POISelect Array": Value Change {
            n174 = event-data() -> ()  [unwired: 1 in, 1 out]
            n175 = disable-structure shown="Disabled" {
              frame Disabled {
                n176 = local read "POISelect Array"() -> (w229:cluster{"System Array":dbl[], "Boolean":bool}[])
                n177 = call "POISelection.vi"("POISelectArrayIn"=w229) -> ("POI array"=w228:dbl[][])  [unwired: 9 in, 1 out]
                n178 = call "ROI entry-Get selected Z-plane index.vi"() -> ("Z-plane selector (index)"=w223:i32)  [unwired: 10 in, 1 out]
                n179 = call "ROI entry-Clear ROI overlay.vi"() -> ("error out"=w226:errorcluster, "Image Out"=w225:T3)  [unwired: 10 in]
                n180 = call "ROI entry-Get Max Proj setting.vi"() -> ("Max Z-projection setting's value"=w224:bool)  [unwired: 10 in, 1 out]
                n181 = for {
                  tunnel: w228 -> [w236] mode=indexing
                  shift-right: [w239] -> w227
                  shift-left: w225 -> [w238]
                  tunnel: w223 -> [w232]
                  tunnel: w226 -> [_]
                  tunnel: w224 -> [w230]
                  n182 = Index Array(array=w236, index=3) -> (element=w234:dbl)
                  n183 = Equal?(x=w234, y=w232) -> (x = y?=w233:bool)
                  n184 = Delete From Array(array=w236, index=0) -> (deleted portion=w231:dbl, array with subset deleted=w237:dbl[])  [unwired: 1 in]
                  n185 = case shown="False" w230 {
                    tunnel: [w245 w256] -> w239
                    tunnel: w238 -> [w244 w255]
                    tunnel: w237 -> [w243 w254]
                    tunnel: w233 -> [w242 _]
                    tunnel: w231 -> [w241 w253]
                    frame False {
                      n186 = case shown="True" w242 {
                        tunnel: [w246 w251] -> w245
                        tunnel: w244 -> [w246 w250]
                        tunnel: w241 -> [_ w249]
                        tunnel: w243 -> [_ w247]
                        frame False {
                        }
                        frame True {
                          n187 = Increment(x=w249) -> (x+1=w248:dbl)
                          n188 = call "PointOverlayV1.vi"("Point"=w247, "Count"=w248, "Image1"=w250) -> ("Image1 Out"=w251:T3)  [unwired: 8 in]
                        }
                      }
                    }
                    frame True {
                      n189 = Increment(x=w253) -> (x+1=w252:dbl)
                      n190 = call "PointOverlayV1.vi"("Point"=w254, "Count"=w252, "Image1"=w255) -> ("Image1 Out"=w256:T3)  [unwired: 8 in]
                    }
                  }
                }
                n191 = call "ROI entry-Image display write.vi"("Value"=w227) -> ()  [unwired: 4 in, 1 out]
              }
              frame Enabled {
              }
            }
          }
          event "Acquisition", "Live Imaging", "Done/Close": Value Change {
            n192 = event-data() -> ("CtlRef"=w259:refnum<vi>)  [unwired: 1 in]
            n193 = call "ROI entry-Event handler-Completion.vi"("Ctrl ref of the control that caused the user event"=w259) -> ("Exit"=w257:bool, "Imaging Mode"=w258:T6)  [unwired: 9 in]
          }
          event "Scan dwell time per pixel (us)", "Trial Length (sec)": Value Change {
            # "Adjusts the Experiment Time and Cool-down time value to the theoretical calculated values which result from the fact that the acquisition time is always an integer multiple of the cycle time."
            n194 = event-data() -> ()  [unwired: 1 in, 1 out]
            n195 = call "Limit entered trial length.vi"() -> ("error out"=w260:errorcluster)  [unwired: 11 in]
            n196 = call "ROI entry screen-Adjust to correct times.vi"("error in (no error)"=w260) -> ()  [unwired: 9 in, 2 out]
          }
          event "Load Reference Image": Value Change {
            # "This button is needed in the ROI entry screen because the equivalent button in the main software panel is disabled while the ROI screen is open (to prevent certain errors which could otherwise occur due to unhandled combinations of UI interaction)."
            n197 = event-data() -> ()  [unwired: 1 in, 1 out]
            n198 = flat-sequence {
              tunnel: [w262] -> w261
              tunnel: w261 -> [w263]
              frame #0 {
                n199 = global read "General Globals.vi" "Movement Correction"() -> (w262:bool)
              }
              frame #1 {
                n200 = call "Event handler-Load ref image.vi"() -> ("error out"=w266:errorcluster, "Error or cancelled"=w265:bool)  [unwired: 10 in]
                n201 = Compound Arithmetic op=OR(w265, w266) -> (w264:bool)
                n202 = case shown="False" w264 {
                  tunnel: w263 -> [w267 _]
                  frame False {
                    # "Ref selected"
                    n203 = case shown="False" w267 {
                      frame False {
                        # "MC was OFF"
                        n204 = global read "gl_ROI Entry UI globals.vi" "ROI entry ctrl refs"() -> (w271:T16)
                        n205 = Unbundle By Name(w271) -> ("Acquisition button"=w272:refnum<vi>)
                        n206 = property on="Property Node" class="Bool"(reference=w272, "DisabledEnum"=2) -> (error out=w268:errorcluster)  [unwired: 1 in, 1 out]
                        n207 = call "fgv_Enforce AOL Z repeat.vi"("Function"=Read_Write_Enum."Write", "Enforce AOL Z repeat"=TRUE) -> ()  [unwired: 8 in, 2 out]
                        n208 = flat-sequence {
                          tunnel: w268 -> [_]
                          frame #0 {
                            n209 = call "Message Window.vi"("Message string"="NOTE\nMovement correction has been automatically enabled.\n\nRepeat the AOL Z-stack with movement correction before you can proceed to functional acquisition.\n") -> ()  [unwired: 10 in, 1 out]
                          }
                        }
                      }
                      frame True {
                      }
                    }
                  }
                  frame True {
                    # "Cancelled or error"
                  }
                }
              }
            }
          }
          event "Enable funct. stimulus", "Funct stim.trig.delay (sec)": Value Change {
            n210 = event-data() -> ()  [unwired: 1 in, 1 out]
            n211 = flat-sequence {
              frame #0 {
                # "Prevents entering trigger delays <1ms"
                n212 = Greater Or Equal?(x="Funct stim.trig.delay (sec)", y=0.001) -> (x >= y?=w277:bool)
                n213 = Select(t="Funct stim.trig.delay (sec)", s=w277, f=0.0) -> (s? t:f=w276:dbl)
                n214 = local write "Funct stim.trig.delay (sec)"(w276) -> ()
              }
              frame #1 {
                n215 = call "Stimulus trigger delay event handler.vi"() -> ()  [unwired: 12 in]
              }
            }
          }
          event "Cool-down time (s)", "Enable cool-down time": Value Change {
            # "Adjusts the Experiment Time and Cool-down time value to the theoretical calculated values which result from the fact that the acquisition time is always an integer multiple of the cycle time."
            n216 = event-data() -> ()  [unwired: 1 in, 1 out]
            n217 = call "ROI entry screen-Adjust to correct times.vi"() -> ()  [unwired: 10 in, 2 out]
          }
          event "Funct stim.trig.delay (sec)", "Enable funct. stimulus": Mouse Enter {
            # "Stops the \"Stimulus trigger delay\" control blinking if blinking was triggered."
            n218 = event-data() -> ()  [unwired: 1 in, 1 out]
            n219 = call "ROI entry-Stop trig delay blinking.vi"() -> ()  [unwired: 12 in]
          }
          event Panel Close {
            w280 = TRUE ("Stop loop")
            n220 = event-data() -> ()  [unwired: 1 in, 1 out]
          }
        }
      }
      frame True {
        # "Initialisation"
        n221 = flat-sequence {
          tunnel: w282 -> [w322]
          tunnel: [w322] -> w281
          tunnel: w281 -> [w328]
          tunnel: [w329] -> w283
          frame #0 {
            n222 = control-ref of="Image Display"() -> (w305:refnum<vi>)
            n223 = control-ref of="Z-Plane Selector"() -> (w302:refnum<vi>)
            n224 = control-ref of="Done/Close"() -> (w293:refnum<vi>)
            n225 = control-ref of="Live Imaging"() -> (w294:refnum<vi>)
            n226 = control-ref of="Acquisition"() -> (w295:refnum<vi>)
            n227 = control-ref of="Equal size"() -> (w300:refnum<vi>)
            n228 = control-ref of="Arb Plane Entry"() -> (w307:refnum<vi>)
            n229 = control-ref of="Whole plane"() -> (w319:refnum<vi>)
            n230 = control-ref of="Clear Last"() -> (w308:refnum<vi>)
            n231 = control-ref of="Clear All"() -> (w309:refnum<vi>)
            n232 = control-ref of="Max Z Proj"() -> (w315:refnum<vi>)
            n233 = control-ref of="Enable funct. stimulus"() -> (w290:refnum<vi>)
            n234 = control-ref of="Enable cool-down time"() -> (w288:refnum<vi>)
            n235 = control-ref of="Load Reference Image"() -> (w284:refnum<vi>)
            n236 = control-ref of="POI dwell time (us)"() -> (w296:refnum<vi>)
            n237 = control-ref of="Scan dwell time per pixel (us)"() -> (w297:refnum<vi>)
            n238 = control-ref of="# of planes"() -> (w298:refnum<vi>)
            n239 = control-ref of="Zoom"() -> (w299:refnum<vi>)
            n240 = control-ref of="Number of lines left"() -> (w303:refnum<vi>)
            n241 = control-ref of="Trial Length (sec)"() -> (w310:refnum<vi>)
            n242 = control-ref of="# POI"() -> (w313:refnum<vi>)
            n243 = control-ref of="Zplane ind"() -> (w316:refnum<vi>)
            n244 = control-ref of="Wavelength (nm)"() -> (w318:refnum<vi>)
            n245 = control-ref of="Number of Trials"() -> (w320:refnum<vi>)
            n246 = control-ref of="Funct stim.trig.delay (sec)"() -> (w321:refnum<vi>)
            n247 = control-ref of="Cool-down time (s)"() -> (w289:refnum<vi>)
            n248 = control-ref of="Motor Z ind. (um)"() -> (w287:refnum<vi>)
            n249 = control-ref of="AOL Z ind. (um)"() -> (w286:refnum<vi>)
            n250 = control-ref of="Channel"() -> (w301:refnum<vi>)
            n251 = control-ref of="Palette Type"() -> (w311:refnum<vi>)
            n252 = control-ref of="Line Mode"() -> (w317:refnum<vi>)
            n253 = control-ref of="ROI move mode"() -> (w291:refnum<vi>)
            n254 = control-ref of="Z-stack folder path"() -> (w304:refnum<vi>)
            n255 = control-ref of="POI Density"() -> (w306:refnum<vi>)
            n256 = control-ref of="Intensity slider"() -> (w312:refnum<vi>)
            n257 = control-ref of="Step size (µm)"() -> (w292:refnum<vi>)
            n258 = Bundle By Name(cluster=T16 {"Done button"=refnum, "Imaging button"=refnum, "Acquisition button"=refnum, "POI dwell time (us)"=refnum, "Scan dwell time per pixel (us)"=refnum, "# of planes"=refnum, "Zoom Ctrl"=refnum, "Equal size"=refnum, "Channel"=refnum, "Image Display"=refnum, "Z-Plane Selector"=refnum, "Number of lines left"=refnum, "Z-stack folder path"=refnum, "POI Density"=refnum, "Arb Plane Entry"=refnum, "Whole plane"=refnum, "Clear Last"=refnum, "Clear All"=refnum, "Trial Length (sec)"=refnum, "Palette Type"=refnum, "Intensity slider"=refnum, "# POI"=refnum, "Max Z Proj"=refnum, "Zplane ind"=refnum, "Wavelength (nm)"=refnum, "Number of Trials"=refnum, "Funct stim.trig.enable"=refnum, "Funct stim.trig.delay (s)"=refnum, "Line Mode"=refnum, "Step size (µm)"=refnum, "ROI move mode"=refnum, "Cool-down time (s)"=refnum, "Enable cool-down time"=refnum, "Motor Z ind. (um)"=refnum, "AOL Z ind. (um)"=refnum, "Load Reference Image"=refnum, "SubPanel Call"=refnum} ("Ctrl refs cluster"), "Done button"=w293, "Imaging button"=w294, "Acquisition button"=w295, "POI dwell time (us)"=w296, "Scan dwell time per pixel (us)"=w297, "# of planes"=w298, "Zoom Ctrl"=w299, "Equal size"=w300, "Channel"=w301, "Image Display"=w305, "Z-Plane Selector"=w302, "Number of lines left"=w303, "Z-stack folder path"=w304, "POI Density"=w306, "Arb Plane Entry"=w307, "Whole plane"=w319, "Clear Last"=w308, "Clear All"=w309, "Trial Length (sec)"=w310, "Palette Type"=w311, "Intensity slider"=w312, "# POI"=w313, "Max Z Proj"=w315, "Zplane ind"=w316, "Line Mode"=w317, "Wavelength (nm)"=w318, "Number of Trials"=w320, "Funct stim.trig.enable"=w290, "Funct stim.trig.delay (s)"=w321, "Step size (µm)"=w292, "ROI move mode"=w291, "Cool-down time (s)"=w289, "Enable cool-down time"=w288, "Motor Z ind. (um)"=w287, "AOL Z ind. (um)"=w286, "Load Reference Image"=w284) -> (w314:T16)
            n259 = global write "gl_ROI Entry UI globals.vi" "ROI entry ctrl refs"(w314) -> ()
          }
          frame #1 {
            n260 = control-ref of="Pane"() -> (w327:refnum<vi>)
            n261 = control-ref of="Pane 2"() -> (w326:refnum<vi>)
            n262 = Build Array(w327, w326) -> (w325:refnum<vi>[])
            n263 = call "ROI entry-Initialisation.vi"("Pane refs array"=w325, "User Events Cluster"=w328) -> ("Open file dialogue window"=w329:bool)  [unwired: 9 in]
            n264 = call "fgv_Enforce AOL Z repeat.vi"("Function"=Read_Write_Enum."Write", "Enforce AOL Z repeat"=FALSE) -> ()  [unwired: 8 in, 2 out]
          }
        }
      }
    }
  }
  n265 = call "ROI entry-Exit actions.vi"("Imaging Mode"=w8, "Stop loop"=w9, "User Events cluster"=w1) -> ("error out"=w7:errorcluster)  [unwired: 8 in]
  n266 = case shown="False" w9 {
    tunnel: w8 -> [w330 _]
    frame False {
      "Next State" <- w330
    }
    frame True {
    }
  }
  n267 = flat-sequence {
    tunnel: w7 -> [_]
    frame #0 {
      n268 = call "Enable-Disable UI by Z stack.vi"() -> ("Controls refs to enable/disable"=w333:refnum<vi>[])  [unwired: 11 in]
      n269 = call "Enable-Disable UI by Motor Z stack.vi"() -> ("Controls to disable"=w331:refnum<vi>[])  [unwired: 11 in]
      n270 = Request Deallocation(TRUE ("flag")) -> ()
      n271 = local write "Done/Close"(FALSE ("Done/Close")) -> ()
      n272 = Build Array (concatenate)(w333, w331) -> (w332:refnum<vi>[])
      n273 = call "Enable-Disable Encoder UI conditionally.vi"() -> ()  [unwired: 11 in, 1 out]
      n274 = call "Enable-Disable UI Elements.vi"("Enable/Disable"=T13."Enabled", "Ctrl ref's"=w332) -> ()  [unwired: 9 in, 1 out]
    }
  }
